vi "Graveyard - Simple.vi"() -> ()   [LabVIEW 2017]
doc: "A demonstration of burying the Corpse (legacy) at the grave (Diagram Disable Structure). This includes step-by-step instructions for removing the grave and leaving only the Spirit (refactored) code behind with one of two methods: shortcut menu plugin or Quick Drop shortcut plugin."
panel:
  out "Any?":bool
  in  "Input":bool[](array[boolean])=[FALSE, FALSE, FALSE, FALSE, FALSE, FALSE, TRUE, FALSE, FALSE, FALSE]
  # "Overview: Demonstrates using the Graveyard (Bookmark Manager) while working with a grave\nInstructions:\n1. Choose only of the following steps to open the Graveyard:\n    A. Select View->Bookmark Manager from the menu bar. A dialog will appear. Select \"Graveyard\" from the list and click \"OK\".\n    B. Select Tools->Field R&D Services->Eulogy->Graveyard...\n2. When the Graveyard appears, select \"Main Application Instance\" from the drop down menu on the left, i.e. \"Scope\". The \"Graveyard - Simple\" VI should appear in the tree. No graves or zombies should be listed.\n3. Switch to the block diagram and follow the instructions to observe modifications in the Graveyard."
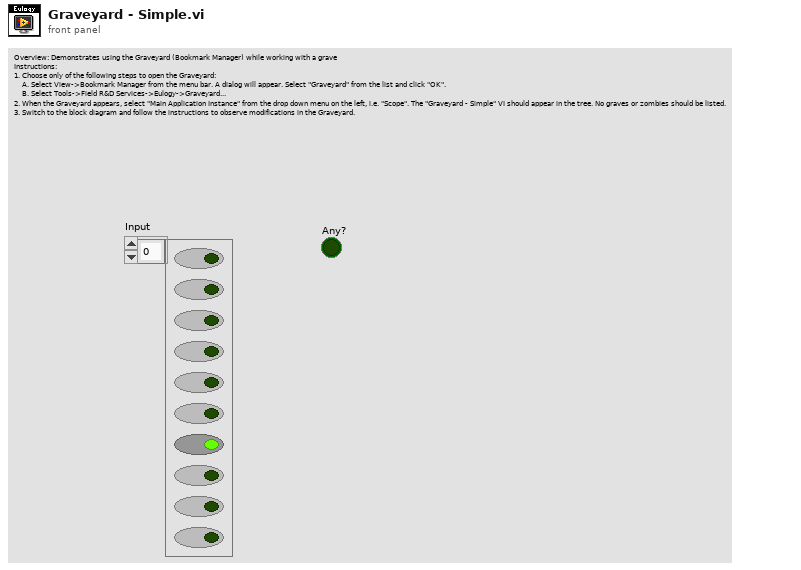
[diagram p1: front panel]
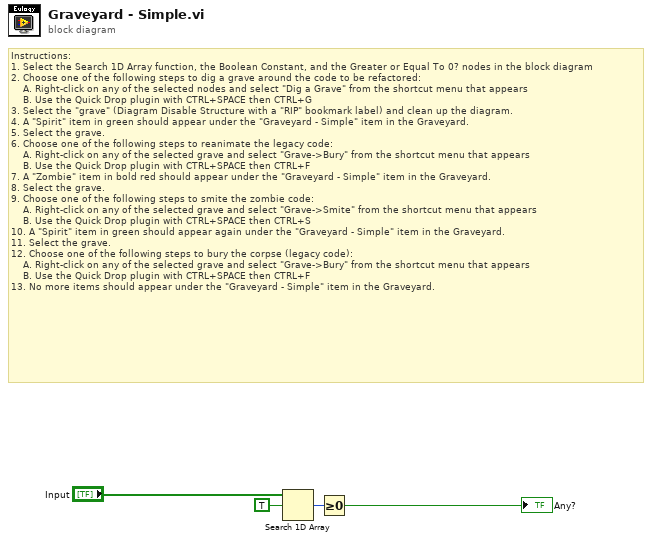
[diagram p0: block diagram]
diagram:
  # "Instructions:\n1. Select the Search 1D Array function, the Boolean Constant, and the Greater or Equal To 0? nodes in the block diagram\n2. Choose one of the following steps to dig a grave around the code to be refactored:\n    A. Right-click on any of the selected nodes and select \"Dig a Grave\" from the shortcut menu that appears\n    B. Use the Quick Drop plugin with CTRL+SPACE then CTRL+G\n3. Select the \"grave\" (Diagram Disable Structure with a \"RIP\" bookmark label) and clean up the diagram. \n4. A \"Spirit\" item in green should appear under the \"Graveyard - Simple\" item in the Graveyard.\n5. Select the grave.\n6. Choose one of the following steps to reanimate the legacy code:\n    A. Right-click on any of the selected grave and select \"Grave->Bury\" from the shortcut menu that appears\n    B. Use the Quick Drop plugin with CTRL+SPACE then CTRL+F\n7. A \"Zombie\" item in bold red should appear under the \"Graveyard - Simple\" item in the Graveyard.\n8. Select the grave.\n9. Choose one of the following steps to smite the zombie code:\n    A. Right-click on any of the selected grave and select \"Grave->Smite\" from the shortcut menu that appears\n    B. Use the Quick Drop plugin with CTRL+SPACE then CTRL+S\n10. A \"Spirit\" item in green should appear again under the \"Graveyard - Simple\" item in the Graveyard.\n11. Select the grave.\n12. Choose one of the following steps to bury the corpse (legacy code):\n    A. Right-click on any of the selected grave and select \"Grave->Bury\" from the shortcut menu that appears\n    B. Use the Quick Drop plugin with CTRL+SPACE then CTRL+F\n13. No more items should appear under the \"Graveyard - Simple\" item in the Graveyard."
  n1 = Search 1D Array(1D array="Input", element=TRUE) -> (index of element=w1:i32)  [unwired: 1 in]
  n2 = Greater Or Equal To 0?(x=w1) -> (x >= 0?=→"Any?":bool)
